vi "Pan_Head.vi"(1 "node":string, 2 "error in":errorcluster, 3 "Speed":dbl, 4 "Target (Degrees)":dbl) -> (0 "error out":errorcluster)   [LabVIEW 2013]
uses:
  <userlib>/ROSforLV/ROS/Code/Console/Servers/ServerSubs/TopicDef.ctl
  <userlib>/ROSforLV/ROS/Code/SubVIs/_ROSDirection.ctl
  <userlib>/ROSforLV/ROS/MessageBuilding/std_msgs/subs/i32Scalar.vi
  <userlib>/ROSforLV/ROS/MessageBuilding/std_msgs/subs/float32Scalar.vi
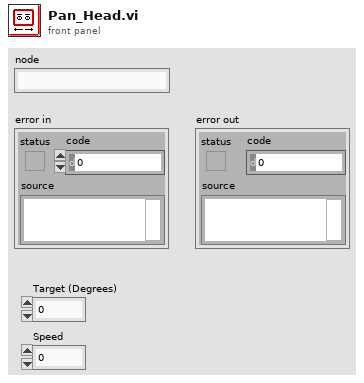
[diagram p1: front panel]
types:
  T1 = typedef "TopicDef.ctl" = cluster{"Topic":string, "Type":string, "Action":T2, "Update (ms)":u16, "write queue":u16}
  T2 = typedef "_ROSDirection.ctl" = enum16{"Node", "Publisher", "Subscriber", "Service Client"}
  T3 = typedef "_ROSControl.ctl" = cluster{"topic port":u16, "Node":string, "topic":string, "type":string, "node port":u32, "error ":errorcluster, "Direction":T2, "APIs":string[], "Update (ms)":u16, "write queue":u16}
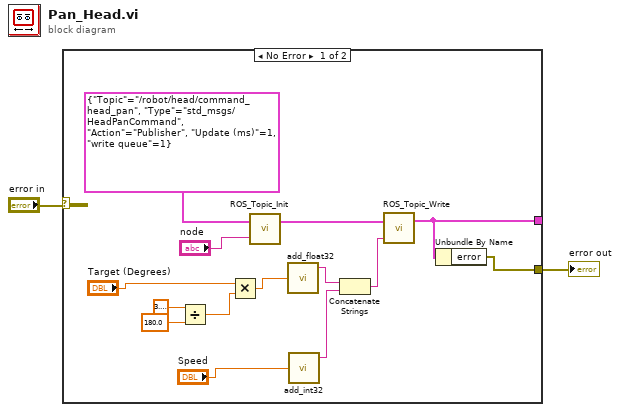
[diagram p0: block diagram]
diagram:
  n1 = case shown="No Error" "error in" {
    selector: "error in" -> [_ w17]
    tunnel: [w13 _] -> _
    tunnel: [w12 w17] -> w1
    frame No Error {
      n2 = Divide(x=3.141592653589793, y=180.0) -> (x/y=w4:dbl)
      n3 = Multiply(x="Target (Degrees)", y=w4) -> (x*y=w3:dbl)
      n4 = call <userlib>:"ROS_Topic_Init.vi"("node"="node", "Definitions"=T1 {"Topic"="/robot/head/command_head_pan", "Type"="std_msgs/HeadPanCommand", "Action"=enum."Publisher", "Update (ms)"=1, "write queue"=1}) -> ("ROS out"=w16:T3)  [unwired: 1 in]
      n5 = call-poly <userlib>:"add_float32.vi"("Numeric"=w3) -> ("msg out"=w10:string)  [unwired: 4 in]
      n6 = call-poly <userlib>:"add_int32.vi"("Numeric"="Speed") -> ("msg out"=w9:string)  [unwired: 4 in]
      n7 = Concatenate Strings(w10, w9) -> (w8:string)
      n8 = call <userlib>:"ROS_Topic_Write.vi"("Msg in"=w8, "ROS in"=w16) -> ("ROS out"=w13:T3)  [unwired: 2 in]
      n9 = Unbundle By Name(w13) -> ("error"=w12:errorcluster)
    }
    frame Error {
    }
  }
  "error out" <- w1
